vi "Nonlinear Curve Fit LM bound.vi"(0 "Y":dbl[](array[numeric]), 1 "f(x,a)":T3, 2 "data":variant, 5 "X":dbl[](array[numeric]), 7 "Weight":dbl[](array[numeric]), 9 "initial parameters":dbl[](array[numeric]), 11 "error in (no error)":errorcluster, 12 "termination":cluster{"max iteration":i32, "tolerance":dbl}={"max iteration"=200, "tolerance"=1e-08}, 13 "parameter bounds":T1, 14 "method":T2 items=["Least Square", "Least Absolute Residual", "Bisquare"]) -> (3 "number of function calls":i32, 4 "best nonlinear fit":dbl[](array[numeric]), 6 "best fit parameters":dbl[](array[numeric]), 8 "covariance":T4, 10 "residue":dbl, 15 "error out":errorcluster)   [LabVIEW 2010, in "NI_Gmath.lvlib"]
doc: "Uses either the Levenberg-Marquardt algorithm or the trust-region dogleg algorithm to determine the set of parameters that best fit the set of input data points (<B>X</B>, <B>Y</B>) as expressed by a nonlinear function y = <B>f(x,a)</B>, where a is the set of parameters. You must manually select the polymorphic instance to use."
uses:
  NI_Gmath.lvlib
  RealMatrix.ctl
  LM model function reference.ctl
  Curve Fitting Criteria.ctl
  stopping criteria.ctl
  LM model function.ctl
  LM_output select.ctl
  Real Inverse Matrix.vi
  NI_AALBase.lvlib
  NI_Matrix.lvlib
  NI_AALPro.lvlib
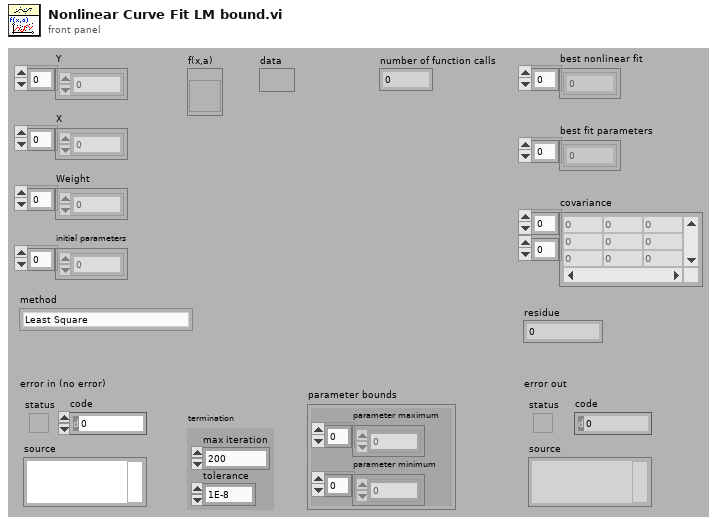
[diagram p1: front panel]
types:
  T1 = cluster{"parameter minimum":dbl[], "parameter maximum":dbl[]}
  T2 = typedef "NI_AALPro.lvlib/Curve Fitting Criteria.ctl" = u16
  T3 = typedef "NI_Gmath.lvlib/LM model function reference.ctl" = refnum<vi>
  T4 = typedef "NI_Matrix.lvlib/RealMatrix.ctl" = dbl[][]
  T5 = typedef "NI_Gmath.lvlib/LM model function.ctl" = cluster{"f(x,a)":T3, "data":variant}
  T6 = typedef "NI_Gmath.lvlib/stopping criteria.ctl" = cluster{"function tolerance":dbl, "parameter tolerance":dbl, "max iterations":i32, "max function calls":i32, "gradient tolerance":dbl, "max time (sec)":dbl}
  T7 = typedef "NI_Gmath.lvlib/stopping criteria with time.ctl" = cluster{"function tolerance":dbl, "parameter tolerance":dbl, "max iterations":i32, "max function calls":i32, "gradient tolerance":dbl, "max time (sec)":dbl, "initial tick count":u32}
  T8 = typedef "NI_Gmath.lvlib/LM_output select.ctl" = cluster{"model function":bool, "gradient":bool}
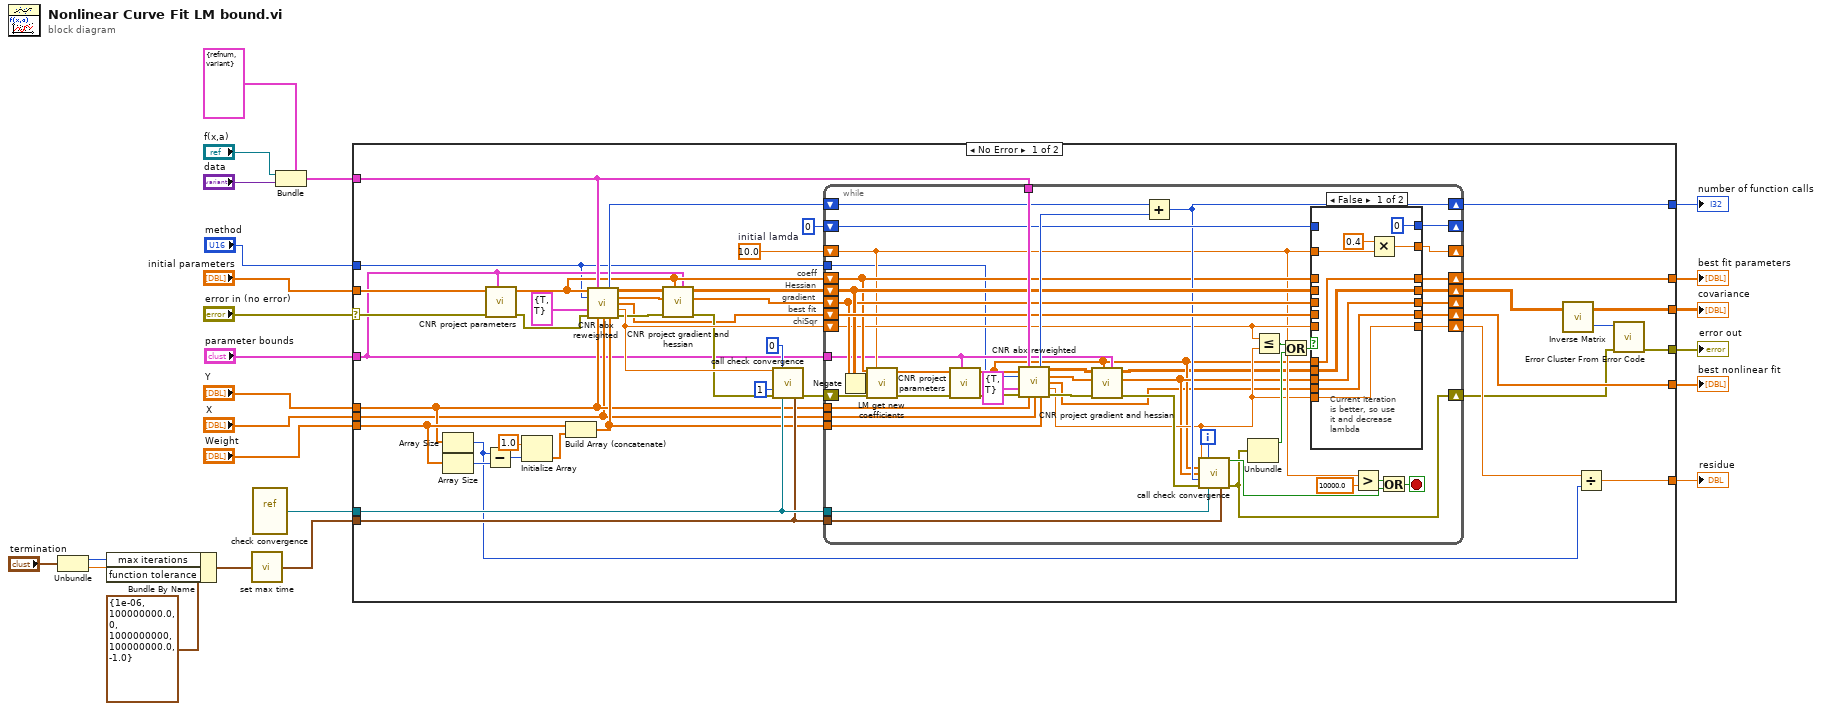
[diagram p0: block diagram]
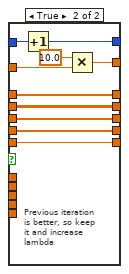
[diagram p2: hidden frame]
diagram:
  n1 = Unbundle("termination") -> ("max iteration"=w12:i32, "tolerance"=w11:dbl)
  n2 = Bundle By Name(cluster=T6 {"function tolerance"=1e-06, "parameter tolerance"=100000000.0, "max iterations"=0, "max function calls"=1000000000, "gradient tolerance"=100000000.0, "max time (sec)"=-1.0} ("stopping criteria"), "max iterations"=w12, "function tolerance"=w11) -> (w4:T6)
  n3 = call "set max time.vi"("stopping criteria"=w4) -> ("stopping criteria"=w3:T7)
  n4 = vi-ref "check convergence.vi"() -> (w10:refnum<vi>)
  n5 = Bundle(cluster=T5 {"f(x,a)"=refnum, "data"=variant} ("model function"), "f(x,a)"="f(x,a)", "data"="data") -> (w6:T5)
  n6 = case shown="No Error" "error in (no error)" {
    selector: "error in (no error)" -> [w37 w136]
    tunnel: [w40 _] -> w24
    tunnel: [w63 _] -> w23
    tunnel: "initial parameters" -> [w38 _]
    tunnel: [w48 _] -> w21
    tunnel: [w61 _] -> w20
    tunnel: "Weight" -> [w57 _]
    tunnel: "Y" -> [w54 _]
    tunnel: w3 -> [w66 _]
    tunnel: "X" -> [w49 _]
    tunnel: [w55 w136] -> w16
    tunnel: w6 -> [w50 _]
    tunnel: w10 -> [w67 _]
    tunnel: [w42 _] -> w9
    tunnel: "method" -> [w25 _]
    tunnel: "parameter bounds" -> [w29 _]
    frame No Error {
      w26 = 10.0  # initial lamda
      # "best fit"
      # "chiSqr"
      # "gradient"
      # "Hessian"
      # "coeff"
      n7 = Array Size(array=w54) -> (size(s)=w39:i32)
      n8 = Array Size(array=w57) -> (size(s)=w60:i32)
      n9 = Subtract(x=w39, y=w60) -> (x-y=w59:i32)
      n10 = call "CNR project parameters.vi"("bounds"=w29, "error in"=w37, "parameters"=w38) -> ("error out"=w36:errorcluster, "projected parameters"=w30:dbl[])  [unwired: 7 out]
      n11 = Initialize Array(1.0, w59) -> (w58:dbl[])
      n12 = Build Array (concatenate)(w57, w58) -> (w65:dbl[])
      n13 = call "CNR abx reweighted.vi"("parameters"=w30, "model function"=w50, "method"=w25, "output control"=T8 {"model function"=TRUE, "gradient"=TRUE}, "error in (no error)"=w36, "Y"=w54, "X"=w49, "Weight"=w65) -> ("number of function calls"=w51:i32, "Hessian"=w33:T4, "gradient"=w32:dbl[], "best fit"=w31:dbl[], "chiSqr"=w53:dbl, "error out"=w35:errorcluster)  [unwired: 1 in, 1 out]
      n14 = call "CNR project gradient and hessian.vi"("bounds"=w29, "projected parameters"=w30, "error in"=w35, "gradient"=w32, "Hessian"=w33) -> ("error out"=w34:errorcluster, "projected gradient"=w27:dbl[], "projected Hessian"=w28:T4)  [unwired: 1 in, 3 out]
      n15 = call "call check convergence.vi"("f"=w53, "current iteration"=0, "number of function evaluations"=1, "error in"=w34, "vi reference"=w67, "stopping criteria"=w66) -> ("error out"=w52:errorcluster)  [unwired: 2 in, 7 out]
      n16 = while {
        tunnel: w49 -> [w110]
        tunnel: w54 -> [w111]
        tunnel: w65 -> [w109]
        shift-left: w53 -> [w86]
        shift-right: [w85] -> w64
        shift-left: w27 -> [w103]
        shift-right: [w114] -> _
        shift-left: w28 -> [w104]
        shift-right: [w115] -> w44
        shift-left: w30 -> [w87]
        shift-right: [w88] -> w40
        shift-left: w26 -> [w84]
        shift-right: [w112] -> _
        shift-right: [w89] -> w47
        shift-left: w52 -> [w113]
        tunnel: w50 -> [w108]
        tunnel: w67 -> [w95]
        tunnel: w66 -> [w94]
        shift-right: [w96] -> w42
        shift-left: w51 -> [w107]
        shift-right: [w105] -> w48
        shift-left: w31 -> [w106]
        shift-right: [w98] -> _
        shift-left: 0 -> [w99]
        tunnel: w25 -> [w69]
        tunnel: w29 -> [w75]
        i -> [w97]
        stop <- w90 stop-if-true
        n17 = Negate(x=w103) -> (-x=w68:dbl[])
        n18 = call "LM get new coefficients.vi"("Coefficients"=w87, "lamda"=w84, "Alpha"=w104, "Beta"=w68, "error in (no error)"=w113) -> ("New Coefficients"=w81:dbl[], "error out"=w83:errorcluster)  [unwired: 9 out]
        n19 = call "CNR project parameters.vi"("bounds"=w75, "error in"=w83, "parameters"=w81) -> ("error out"=w82:errorcluster, "projected parameters"=w74:dbl[])  [unwired: 7 out]
        n20 = call "CNR abx reweighted.vi"("parameters"=w74, "model function"=w108, "method"=w69, "output control"=T8 {"model function"=TRUE, "gradient"=TRUE}, "error in (no error)"=w82, "Y"=w111, "X"=w110, "Weight"=w109) -> ("number of function calls"=w116:i32, "Hessian"=w73:T4, "gradient"=w77:dbl[], "best fit"=w71:dbl[], "chiSqr"=w78:dbl, "error out"=w80:errorcluster)  [unwired: 1 in, 1 out]
        n21 = call "CNR project gradient and hessian.vi"("bounds"=w75, "projected parameters"=w74, "error in"=w80, "gradient"=w77, "Hessian"=w73) -> ("error out"=w79:errorcluster, "projected gradient"=w76:dbl[], "projected Hessian"=w72:T4)  [unwired: 1 in, 3 out]
        n22 = Add(x=w107, y=w116) -> (x+y=w96:i32)
        n23 = call "call check convergence.vi"("f"=w78, "current iteration"=w97, "X"=w74, "gradient"=w76, "number of function evaluations"=w96, "error in"=w79, "vi reference"=w95, "stopping criteria"=w94) -> ("stop?"=w92:bool, "error out"=w89:errorcluster)  [unwired: 6 out]
        n24 = Unbundle(w89) -> ("status"=w101:bool)  [unwired: 2 out]
        n25 = Less Or Equal?(x=w86, y=w78) -> (x <= y?=w102:bool)
        n26 = Or(x=w102, y=w101) -> (x .or. y?=w100:bool)
        n27 = case shown="False" w100 {
          tunnel: [w122 w135] -> w115
          tunnel: w104 -> [_ w135]
          tunnel: [w121 w134] -> w114
          tunnel: w74 -> [w118 _]
          tunnel: w103 -> [_ w134]
          tunnel: w87 -> [_ w133]
          tunnel: [w118 w133] -> w88
          tunnel: [w123 w129] -> w112
          tunnel: w86 -> [_ w132]
          tunnel: w78 -> [w119 _]
          tunnel: [w119 w132] -> w85
          tunnel: w84 -> [w125 w130]
          tunnel: w72 -> [w122 _]
          tunnel: w76 -> [w121 _]
          tunnel: w106 -> [_ w128]
          tunnel: w71 -> [w120 _]
          tunnel: [w120 w128] -> w105
          tunnel: w99 -> [_ w127]
          tunnel: [0 w126] -> w98
          frame False {
            # "Current iteration\nis better, so use\nit and decrease \nlambda"
            n28 = Multiply(x=0.4, y=w125) -> (x*y=w123:dbl)
          }
          frame True {
            # "Previous iteration\nis better, so keep\nit and increase \nlambda"
            n29 = Increment(x=w127) -> (x+1=w126:i32)
            n30 = Multiply(x=10.0, y=w130) -> (x*y=w129:dbl)
          }
        }
        n31 = Greater?(x=w84, y=10000.0) -> (0:w91:bool)
        n32 = Or(x=w91, y=w92) -> (x .or. y?=w90:bool)
      }
      n33 = call-poly "Inverse Matrix.vi"("Input Matrix"=w44) -> ("error"=w56:i32, "Inverse Matrix"=w61:T4)  [unwired: 1 in]
      n34 = Divide(x=w64, y=w39) -> (x/y=w63:dbl)
      n35 = call "Error Cluster From Error Code.vi"("error in (no error)"=w47, "error code (0)"=w56) -> ("error out"=w55:errorcluster)  [unwired: 1 in, 6 out]
    }
    frame Error {
    }
  }
  "residue" <- w23
  "best fit parameters" <- w24
  "best nonlinear fit" <- w21
  "error out" <- w16
  "covariance" <- w20
  "number of function calls" <- w9
